vi "enumerateStaticDependencies.vi"(8 "error in (no error)":errorcluster, 11 "Instrument":refnum<class "Instrument.lvclass">) -> (0 "error out":errorcluster, 2 "Static Dependencies":refnum<class "Dependency.lvclass">[](array[class]), 3 "Instrument out":refnum<class "Instrument.lvclass">)   [LabVIEW 2020, in "Instrument.lvclass"]
doc: "JKI State Machine Objects (SMO) 1.3.0.56\nJKI - JKI\nCopyright (c) 2017, JKI"
uses:
  Instrument.lvclass
  C:/Program Files (x86)/National Instruments/LabVIEW 2020/vi.lib/JKI/JKI SMO/SMO/SMO.lvclass
  <vilib>/JKI/JKI SMO/Dependency/Dependency.lvclass
  RemoteControl/RemoteControl.lvclass
  RemoteControl.STM/RemoteControl.STM.lvclass
  C:/Users/gsa/Documents/GitHub/Instrument-Framework/lvsrc/SMOs/RemoteControl/RemoteControl.lvclass
  Logger.DSC/Logger.DSC.lvclass
  <vilib>/Utility/sysdir.llb/System Directory Type.ctl
  Logger.Error/Logger.Error.lvclass
  Instrument.lvclass/Instrument.ctl
  RemoteControl/RemoteControl.lvclass/RemoteControl.ctl
  LevyLab/LevyLab.lvclass
  <vilib>/JKI/JKI SMO/SMO/SMO.lvclass
panel:
  # "For instructions on how to use the JKI State Machine Objects, examples and video tutorials, visit:\nhttp://jki.net/state-machine-objects/\n\nJKI State Machine Objects™\nhttp://jki.net/state-machine-objects/\nCopyright (C) 2005-2015, JKI <info@jki.net>\nALL RIGHTS RESERVED"
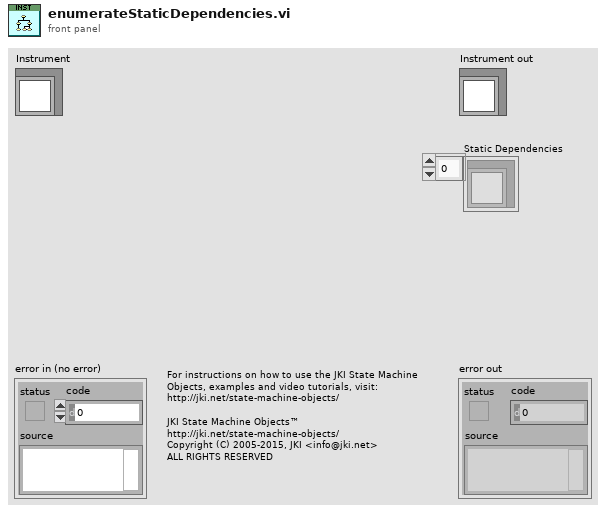
[diagram p1: front panel]
types:
  T1 = typedef "System Directory Type.ctl" = i32
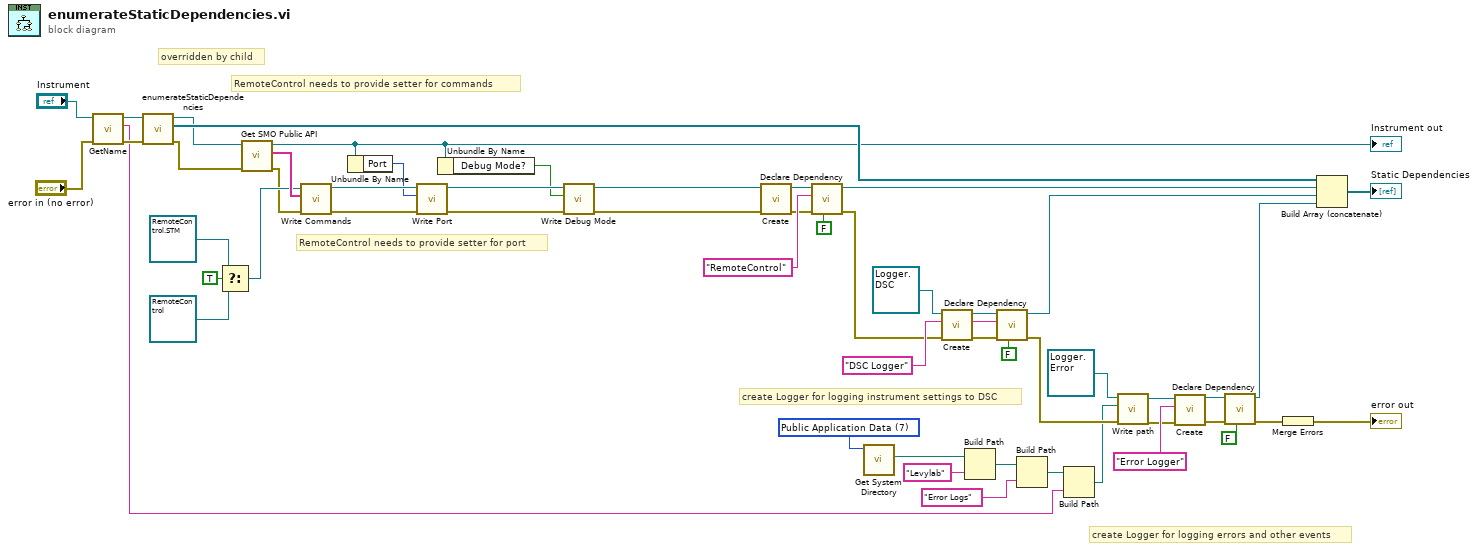
[diagram p0: block diagram]
diagram:
  w38 = T1 7 items=["User Home"=0, "User Desktop"=1, "User Documents"=2, "User Application Data"=3, "User Preferences"=4, "User Temporary"=5, "Public Documents"=6, "Public Application Data"=7, "Public Preferences"=8, "Public Cache"=13, "System Core Libraries"=9, "System Installed Libraries"=10, "Application Files"=11, "Boot Volume Root"=12] ("system directory type")
  # "create Logger for logging errors and other events"
  # "create Logger for logging instrument settings to DSC"
  # "RemoteControl needs to provide setter for port"
  # "RemoteControl needs to provide setter for commands"
  # "overridden by child"
  n1 = call <vilib>:"GetName.vi"("error in (no error)"="error in (no error)", "SMO"="Instrument") -> ("error out"=w33:errorcluster, "Name"=w5:string, "SMO out"=w34:refnum<class "Instrument.lvclass">)  [unwired: 7 in]
  n2 = call-parent "enumerateStaticDependencies.vi"("error in (no error)"=w33, "SMO"=w34) -> ("error out"=w23:errorcluster, "Static Dependencies"=w53:refnum<class "Dependency.lvclass">[], "SMO out"=w45:refnum<class "Instrument.lvclass">)  [unwired: 7 in]
  n3 = Select(t=refnum<class "RemoteControl.STM.lvclass"> refnum ("RemoteControl.STM.lvclass"), s=TRUE, f=refnum<class "RemoteControl.lvclass"> refnum ("RemoteControl.lvclass")) -> (s? t:f=w12:refnum<class "RemoteControl.lvclass">)
  n4 = call-dynamic "Get SMO Public API.vi"("error in (no error)"=w23, "Instrument in"=w45) -> ("error out"=w2:errorcluster, "Commands"=w13:string[], "Instrument out"=w3:refnum<class "Instrument.lvclass">)  [unwired: 7 in]
  "Instrument out" <- w3
  n5 = call-dynamic "Write Commands.vi"("error in (no error)"=w2, "Commands"=w13, "RemoteControl in"=w12) -> ("error out"=w24:errorcluster, "RemoteControl out"=w50:refnum<class "RemoteControl.lvclass">)  [unwired: 7 in]
  n6 = Unbundle By Name(w3) -> ("Port"=w4:u16)
  n7 = call-dynamic "Write Port.vi"("error in (no error)"=w24, "Port"=w4, "RemoteControl in"=w50) -> ("error out"=w11:errorcluster, "RemoteControl out"=w9:refnum<class "RemoteControl.lvclass">)  [unwired: 7 in]
  n8 = Unbundle By Name(w3) -> ("Debug Mode?"=w1:bool)
  n9 = call "Write Debug Mode.vi"("error in (no error)"=w11, "Debug Mode?"=w1, "RemoteControl in"=w9) -> ("error out"=w10:errorcluster, "RemoteControl out"=w8:refnum<class "RemoteControl.lvclass">)  [unwired: 7 in]
  n10 = call <vilib>:"Create.vi"("error in (no error)"=w10, "SMO"=w8) -> ("error out"=w14:errorcluster, "SMO out"=w15:refnum<class "RemoteControl.lvclass">)  [unwired: 7 in, 1 out]
  n11 = call <vilib>:"Declare Dependency.vi"("Shared Resource (F)"=FALSE, "error in (no error)"=w14, "Name"="RemoteControl", "Type"=w15) -> ("error out"=w42:errorcluster, "Dependency out"=w54:refnum<class "Dependency.lvclass">)  [unwired: 6 in]
  n12 = call <vilib>:"Get System Directory.vi"("system directory type"=w38) -> ("system directory"=w40:path)  [unwired: 10 in]
  n13 = call <vilib>:"Create.vi"("error in (no error)"=w42, "Subsystem Name (optional)"="DSC Logger" ("Name"), "SMO"=refnum<class "Logger.DSC.lvclass"> refnum ("Logger.DSC.lvclass")) -> ("error out"=w47:errorcluster, "SMO name"=w43:string, "SMO out"=w48:refnum<class "Logger.DSC.lvclass">)  [unwired: 6 in]
  n14 = Build Path(base path=w40, name or relative path="Levylab") -> (appended path=w29:path)
  n15 = call <vilib>:"Declare Dependency.vi"("Shared Resource (F)"=FALSE, "error in (no error)"=w47, "Name"=w43, "Type"=w48) -> ("error out"=w20:errorcluster, "Dependency out"=w37:refnum<class "Dependency.lvclass">)  [unwired: 6 in]
  n16 = Build Path(base path=w29, name or relative path="Error Logs") -> (appended path=w7:path)
  n17 = Build Path(base path=w7, name or relative path=w5) -> (appended path=w6:path)
  n18 = call-dynamic "Write path.vi"("error in (no error)"=w20, "path"=w6, "Logger in"=refnum<class "Logger.Error.lvclass"> refnum ("Logger.Error.lvclass")) -> ("error out"=w18:errorcluster, "Logger out"=w19:refnum<class "Logger.Error.lvclass">)  [unwired: 7 in]
  n19 = call <vilib>:"Create.vi"("error in (no error)"=w18, "Subsystem Name (optional)"="Error Logger" ("Name"), "SMO"=w19) -> ("error out"=w16:errorcluster, "SMO out"=w17:refnum<class "Logger.Error.lvclass">)  [unwired: 6 in, 1 out]
  n20 = call <vilib>:"Declare Dependency.vi"("Shared Resource (F)"=FALSE, "error in (no error)"=w16, "Type"=w17) -> ("error out"=w30:errorcluster, "Dependency out"=w31:refnum<class "Dependency.lvclass">)  [unwired: 7 in]
  n21 = Merge Errors(w30) -> (→"error out":errorcluster)
  n22 = Build Array (concatenate)(w53, w54, w37, w31) -> (→"Static Dependencies":refnum<class "Dependency.lvclass">[])
